vi "set_jog_step.vi"(6 "Motor \"Name\"":string="1", 7 "error in (no error)":errorcluster, 8 "Encoder Pulses per Degree":i32=398, 9 "Degrees":dbl, 10 "VISA resource name":refnum<visa-resource-name>="COM3") -> (0 "error out":errorcluster, 3 "VISA resource name out":refnum<visa-resource-name>)   [LabVIEW 2024]
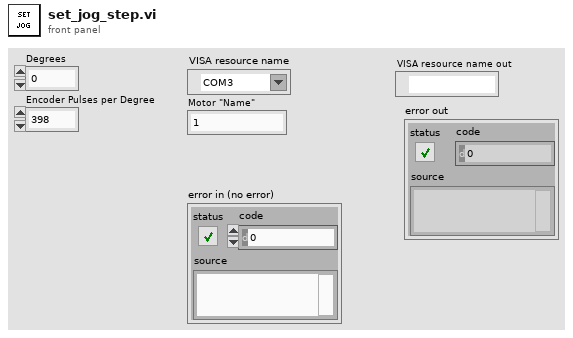
[diagram p1: front panel]
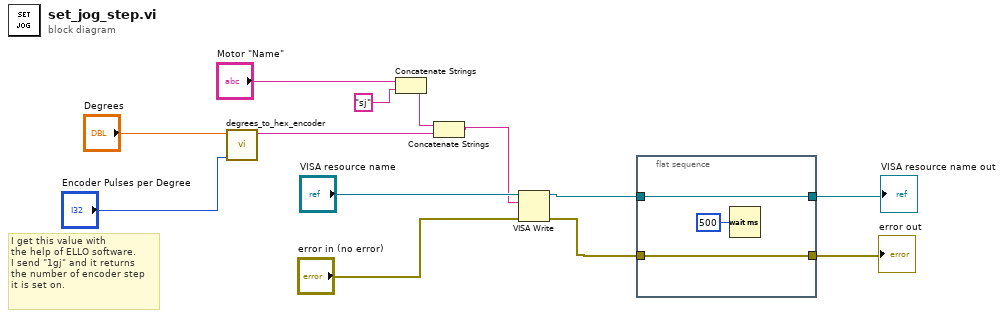
[diagram p0: block diagram]
diagram:
  # "I get this value with\nthe help of ELLO software.\nI send \"1gj\" and it returns\nthe number of encoder step\nit is set on."
  n1 = call "degrees_to_hex_encoder.vi"("Encoder Pulses per Degree"="Encoder Pulses per Degree", "Degrees"="Degrees") -> ("hex integer string"=w1:string)  [unwired: 8 in, 1 out]
  n2 = Concatenate Strings("Motor \"Name\"", "sj" ("string")) -> (w9:string)
  n3 = Concatenate Strings(w9, w1) -> (w8:string)
  n4 = VISA Write(VISA resource name="VISA resource name", write buffer=w8, error in (no error)="error in (no error)") -> (VISA resource name out=w6:refnum<visa-resource-name>, error out=w4:errorcluster)  [unwired: 1 out]
  n5 = flat-sequence {
    tunnel: [w16] -> w7
    tunnel: w6 -> [w16]
    tunnel: [w15] -> w5
    tunnel: w4 -> [w15]
    frame #0 {
      n6 = Wait (ms)(milliseconds to wait=u32 500) -> ()  [unwired: 1 out]
    }
  }
  "error out" <- w5
  "VISA resource name out" <- w7
